vi "Sort 2 1-D arrays.vi"(2 "Array 2":dbl[](array[numeric]) format="%.2f", 3 "Array 1":dbl[](array[numeric]) format="%.2f") -> (0 "Array 2":dbl[](array[numeric]) format="%.2f", 1 "Array 1":dbl[](array[numeric]) format="%.2f")   [LabVIEW 2025]
doc: "This VI will sort two 1 dimensional arrays of double precison numbers. The two arrays are kept in synchronization and sorted in order of the first array values.\nScott Hannahs, <sth@magnet.fsu.edu> NHMFL-FSU, May 2003\nAuthor: Scott Hannahs <sth@magnet.fsu.edu>\n\nThis software is licensed for use under the “MIT License\"\nCopyright (c) 2025 Scott Hannahs, sth@sth@magnet.sthnet.net\n\nPermission is hereby granted, free of charge, to any person obtaining a copy of this software and associated documentation files (the \"Software\"), to deal in the Software without restriction, including without limitation the rights to use, copy, modify, merge, publish, distribute, sublicense, and/or sell copies of the Software, and to permit persons to whom the Software is furnished to do so, subject to the following conditions: The above copyright notice and this permission notice shall be included in all copies or substantial portions of the Software.\n\nTHE SOFTWARE IS PROVIDED \"AS IS\", WITHOUT WARRANTY OF ANY KIND, EXPRESS OR IMPLIED, INCLUDING BUT NOT LIMITED TO THE WARRANTIES OF MERCHANTABILITY, FITNESS FOR A PARTICULAR PURPOSE AND NONINFRINGEMENT. IN NO EVENT SHALL THE AUTHORS OR COPYRIGHT HOLDERS BE LIABLE FOR ANY CLAIM, DAMAGES OR OTHER LIABILITY, WHETHER IN AN ACTION OF CONTRACT, TORT OR OTHERWISE, ARISING FROM, OUT OF OR IN CONNECTION WITH THE SOFTWARE OR THE USE OR OTHER DEALINGS IN THE SOFTWARE."
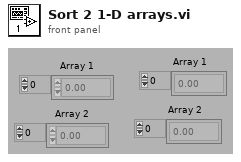
[diagram p1: front panel]
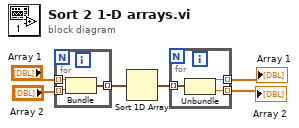
[diagram p0: block diagram]
diagram:
  n1 = for {
    tunnel: "Array 1" -> [w9] mode=indexing
    tunnel: "Array 2" -> [w7] mode=indexing
    tunnel: [w8] -> w4 mode=indexing
    n2 = Bundle(w9, w7) -> (w8:cluster{dbl, dbl})  [unwired: 1 in]
  }
  n3 = Sort 1D Array(array=w4) -> (sorted array=w3:cluster{dbl, dbl}[])
  n4 = for {
    tunnel: w3 -> [w12] mode=indexing
    tunnel: [w11] -> w2 mode=indexing
    tunnel: [w10] -> w1 mode=indexing
    n5 = Unbundle(w12) -> (w11:dbl, w10:dbl)
  }
  "Array 1" <- w2
  "Array 2" <- w1
